vi "Handle Actor Core Events.vi"(8 "error in (no error)":errorcluster, 11 "ActorAutoRegistration in":refnum<class "ActorAutoRegistration.lvclass">) -> (0 "error out":errorcluster, 3 "ActorAutoRegistration out":refnum<class "ActorAutoRegistration.lvclass">)   [LabVIEW 2015, in "ActorAutoRegistration.lvlib" / "ActorAutoRegistration.lvclass"]
uses:
  ActorAutoRegistration.lvclass
  ActorAutoRegistration.lvclass/ActorAutoRegistration.ctl
  ActorAutoRegistration Messages/DBLValueMsg/DBLValueMsg.lvclass
  ActorAutoRegistration Messages/I32ValueMsg/I32ValueMsg.lvclass
  ActorAutoRegistration Messages/BooleanValueMsg/BooleanValueMsg.lvclass
  ActorAutoRegistration Messages/SGLValueMsg/SGLValueMsg.lvclass
  ActorAutoRegistration Messages/U32ValueMsg/U32ValueMsg.lvclass
  ActorAutoRegistration Messages/StringValueMsg/StringValueMsg.lvclass
  ActorAutoRegistration Messages/PanelCloseMsg/PanelCloseMsg.lvclass
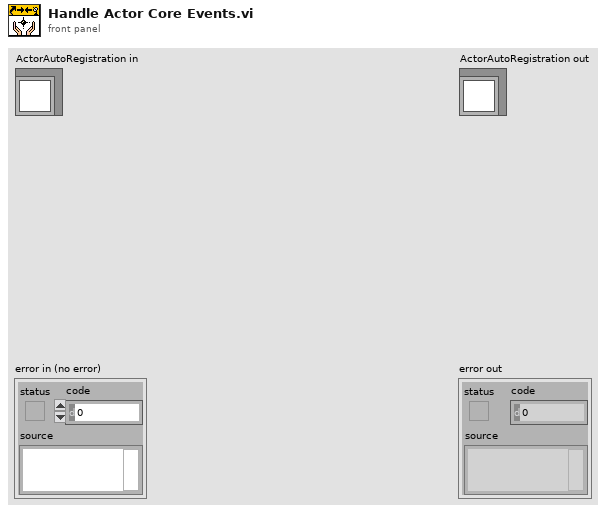
[diagram p1: front panel]
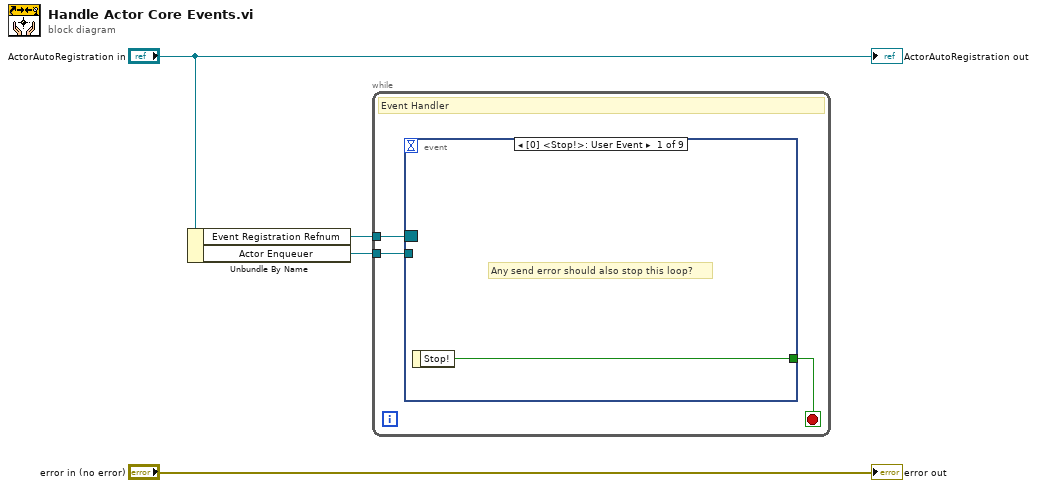
[diagram p0: block diagram]
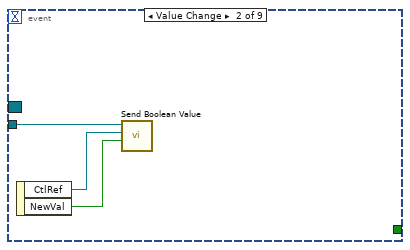
[diagram p2: hidden frame]
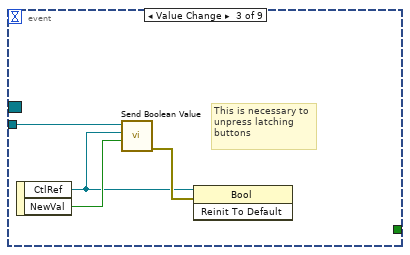
[diagram p3: hidden frame]
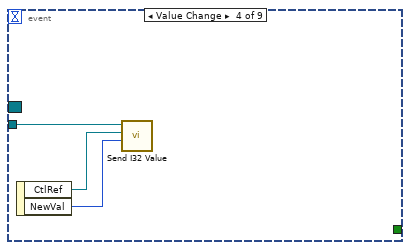
[diagram p4: hidden frame]
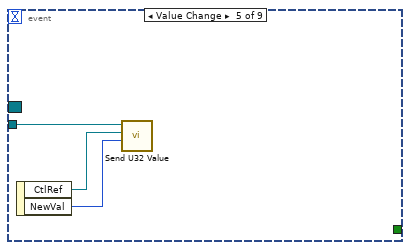
[diagram p5: hidden frame]
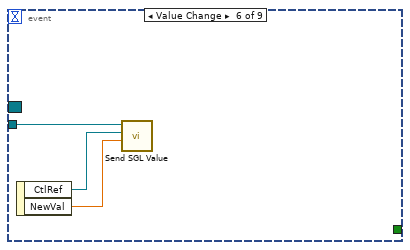
[diagram p6: hidden frame]
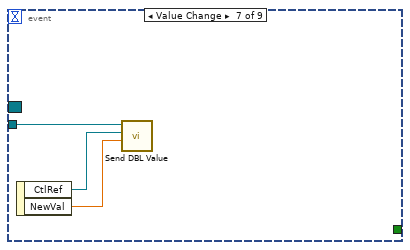
[diagram p7: hidden frame]
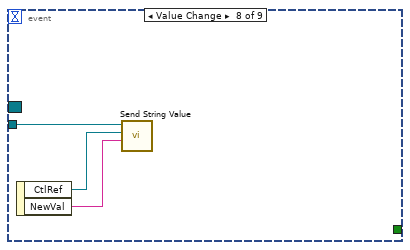
[diagram p8: hidden frame]
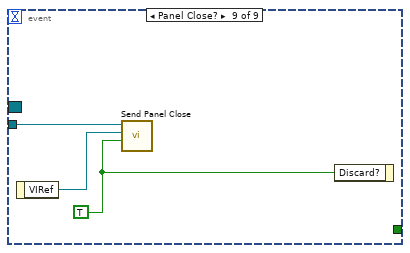
[diagram p9: hidden frame]
diagram:
  n1 = Unbundle By Name("ActorAutoRegistration in") -> ("Event Registration Refnum"=w2:refnum<event-registration>, "Actor Enqueuer"=w1:refnum<class "Message Enqueuer.lvclass">)
  n2 = while {
    tunnel: w2 -> [w7]
    tunnel: w1 -> [w5]
    stop <- w6 stop-if-true
    # "Event Handler"
    n3 = event shown="[0] <Stop!>: User Event" {
      selector: w7 -> [_ _ _ _ _ _ _ _ _]
      dyn-events: _ -> [_ _ _ _ _ _ _ _ _]
      timeout: _ -> [_ _ _ _ _ _ _ _ _]
      tunnel: [w8 _ _ _ _ _ _ _ _] -> w6
      tunnel: w5 -> [_ w9 w14 w16 w19 w22 w25 w28 w33]
      event User Event {
        # "Any send error should also stop this loop?"
        n4 = event-data() -> ("Stop!"=w8:bool)  [unwired: 1 in]
      }
      event Value Change {
        n5 = event-data() -> ("CtlRef"=w11:refnum<vi>, "NewVal"=w10:bool)  [unwired: 1 in]
        n6 = call "Send Boolean Value.vi"("Value"=w10, "Boolean Refnum"=w11, "Message Enqueuer in"=w9) -> ()  [unwired: 8 in, 1 out]
      }
      event Value Change {
        # "This is necessary to\nunpress latching\nbuttons"
        n7 = event-data() -> ("CtlRef"=w12:refnum<vi>, "NewVal"=w15:bool)  [unwired: 1 in]
        n8 = call "Send Boolean Value.vi"("Value"=w15, "Boolean Refnum"=w12, "Message Enqueuer in"=w14) -> ("error out"=w13:errorcluster)  [unwired: 8 in]
        n9 = invoke class="Bool" method="Reinit To Default"(reference=w12, error in=w13) -> ()  [unwired: 1 in, 3 out]
      }
      event Value Change {
        n10 = event-data() -> ("CtlRef"=w18:refnum<vi>, "NewVal"=w17:i32)  [unwired: 1 in]
        n11 = call "Send I32 Value.vi"("Value"=w17, "I32 Refnum"=w18, "Message Enqueuer in"=w16) -> ()  [unwired: 8 in, 1 out]
      }
      event Value Change {
        n12 = event-data() -> ("CtlRef"=w21:refnum<vi>, "NewVal"=w20:u32)  [unwired: 1 in]
        n13 = call "Send U32 Value.vi"("Value"=w20, "U32 Refnum"=w21, "Message Enqueuer in"=w19) -> ()  [unwired: 8 in, 1 out]
      }
      event Value Change {
        n14 = event-data() -> ("CtlRef"=w24:refnum<vi>, "NewVal"=w23:sgl)  [unwired: 1 in]
        n15 = call "Send SGL Value.vi"("Value"=w23, "SGL Refnum"=w24, "Message Enqueuer in"=w22) -> ()  [unwired: 8 in, 1 out]
      }
      event Value Change {
        n16 = event-data() -> ("CtlRef"=w27:refnum<vi>, "NewVal"=w26:dbl)  [unwired: 1 in]
        n17 = call "Send DBL Value.vi"("Value"=w26, "DBL Refnum"=w27, "Message Enqueuer in"=w25) -> ()  [unwired: 8 in, 1 out]
      }
      event Value Change {
        n18 = event-data() -> ("CtlRef"=w30:refnum<vi>, "NewVal"=w29:string)  [unwired: 1 in]
        n19 = call "Send String Value.vi"("Value"=w29, "String Refnum"=w30, "Message Enqueuer in"=w28) -> ()  [unwired: 8 in, 1 out]
      }
      event Panel Close? {
        w31 = TRUE ("Discarded?")
        n20 = event-data() -> ("VIRef"=w32:refnum<vi>)  [unwired: 1 in]
        n21 = call "Send Panel Close.vi"("Discarded?"=w31, "VI Refnum"=w32, "Message Enqueuer in"=w33) -> ()  [unwired: 8 in, 1 out]
        n22 = event-data("Discard?"=w31) -> ()  [unwired: 1 in, 1 out]
      }
    }
  }
  "error out" <- "error in (no error)"
  "ActorAutoRegistration out" <- "ActorAutoRegistration in"
